vi "resize_array.vi"() -> ()   [LabVIEW 2020]
panel:
  in  "Library Path":path=path "/home/saman/src/lvcc/build/test/libtest.so"
  out "error out":errorcluster
  in  "New Size":i32=2
  in  "array":i32[](array[numeric])=[1, 2, 3]
  out "Resized Array":i32[](array[numeric])=[2, 4, 6, 8]
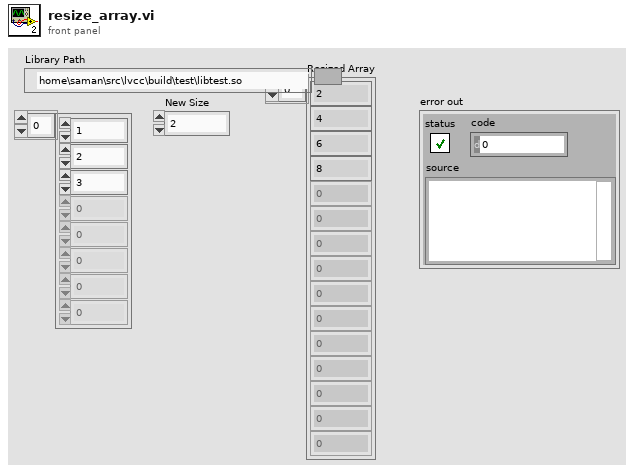
[diagram p1: front panel]
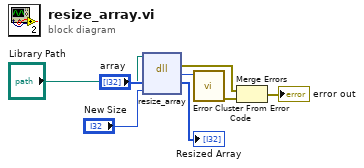
[diagram p0: block diagram]
diagram:
  n1 = dll-call lib="home/saman/src/lvcc/build/test/libtest.so" fn="resize_array"(path in="Library Path", "arr"="array", "size"="New Size") -> (error out=w2:errorcluster, "return type"=w5:i32, "arr"=→"Resized Array":i32[])  [unwired: 3 in, 1 out]
  n2 = call <vilib>:"Error Cluster From Error Code.vi"("error code (0)"=w5) -> ("error out"=w3:errorcluster)  [unwired: 8 in]
  n3 = Merge Errors(w2, w3) -> (→"error out":errorcluster)
